vi "SVI_NewE2E_FindComPort.vi"(2 "Error In":errorcluster, 3 "ID to Match":string) -> (0 "error out":errorcluster, 1 "VISA resource name":refnum<visa-resource-name>)   [LabVIEW 2014]
uses:
  <vilib>/regexp/Match Regular Expression.xnode
panel:
  out "ID Message":string
  out "Responses":string[][](array[string])
  out "Attempts Taken":i32
  out "Current Check":refnum<visa-resource-name>
  out "COM only list":string[](array[string])
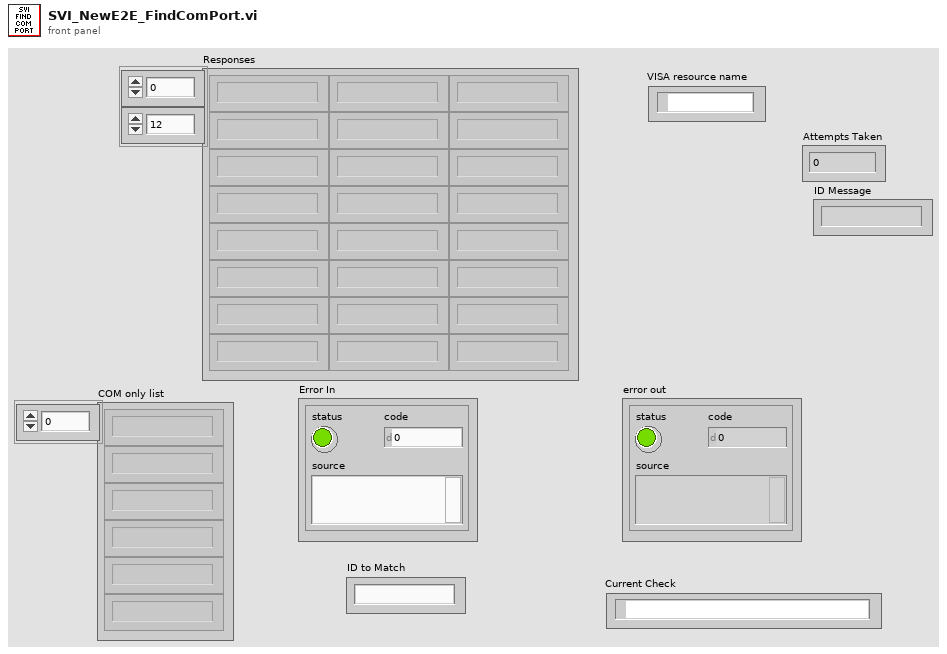
[diagram p1: front panel]
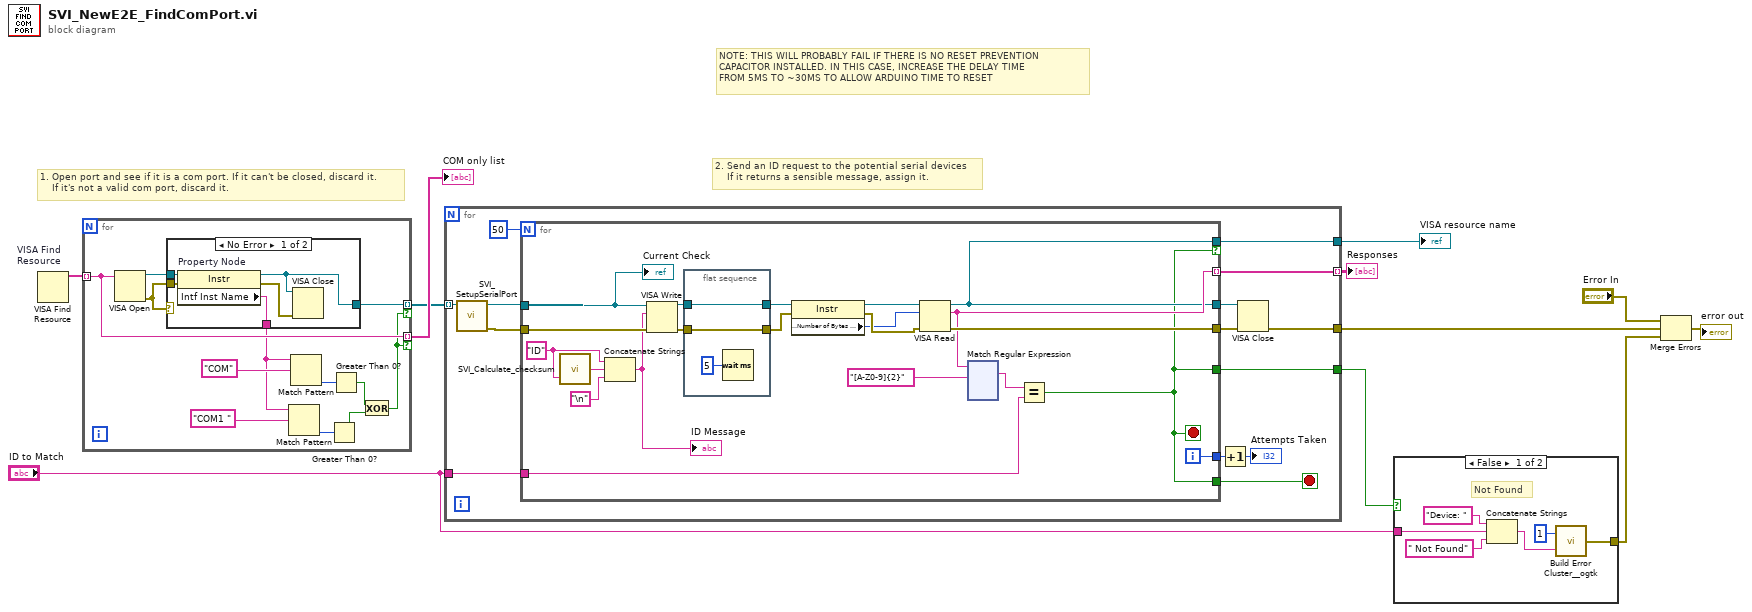
[diagram p0: block diagram]
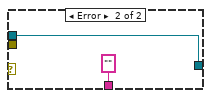
[diagram p2: hidden frame]
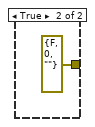
[diagram p3: hidden frame]
diagram:
  # "NOTE: THIS WILL PROBABLY FAIL IF THERE IS NO RESET PREVENTION\nCAPACITOR INSTALLED. IN THIS CASE, INCREASE THE DELAY TIME \nFROM 5MS TO ~30MS TO ALLOW ARDUINO TIME TO RESET"
  # "2. Send an ID request to the potential serial devices\n    If it returns a sensible message, assign it."
  # "1. Open port and see if it is a com port. If it can't be closed, discard it.\n    If it's not a valid com port, discard it."
  n1 = VISA Find Resource "VISA Find\nResource"() -> (3:w11:string[])  [unwired: 3 in, 2 out]
  n2 = for {
    tunnel: w11 -> [w20] mode=indexing
    tunnel: [w20] -> w10 mode=indexing if=w14
    tunnel: [w19] -> w9 mode=indexing if=w14
    n3 = VISA Open(VISA resource name=w20) -> (VISA resource name=w23:refnum<visa-resource-name>, error out=w12:errorcluster)  [unwired: 4 in]
    n4 = case shown="No Error" w12 {
      tunnel: w23 -> [w28 w30]
      tunnel: w12 -> [w27 _]
      tunnel: [w25 w30] -> w19
      tunnel: [w24 "" ("Intf Inst Name")] -> w13
      frame No Error {
        n5 = property on="Property Node" class="Instr"(reference=w28, error in=w27) -> (reference out=w25:refnum<visa-resource-name>, error out=w26:errorcluster, "Intf Inst Name"=w24:string)
        n6 = VISA Close(VISA resource name=w25, error in (no error)=w26) -> ()  [unwired: 1 out]
      }
      frame Error {
      }
    }
    n7 = Match Pattern(string=w13, regular expression="COM1 ") -> (offset past match=w18:i32)  [unwired: 1 in, 3 out]
    n8 = Match Pattern(string=w13, regular expression="COM") -> (offset past match=w21:i32)  [unwired: 1 in, 3 out]
    n9 = Greater Than 0?(x=w18) -> (x > 0?=w16:bool)
    n10 = Greater Than 0?(x=w21) -> (x > 0?=w15:bool)
    n11 = Exclusive Or(1:w16, 2:w15) -> (0:w14:bool)
  }
  "COM only list" <- w10
  n12 = for {
    tunnel: w9 -> [w39] mode=indexing
    tunnel: [w38] -> w5
    tunnel: [w37] -> w3 mode=indexing
    tunnel: [w36] -> w2
    tunnel: "ID to Match" -> [w33]
    tunnel: [w32] -> w8
    stop <- w34 stop-if-true
    n13 = call "SVI_SetupSerialPort.vi"("VISA Refnum in"=w39) -> ("error out"=w40:errorcluster, "VISA Refnum out"=w44:refnum<visa-resource-name>)  [unwired: 9 in]
    n14 = for {
      N: 50 -> [_]
      tunnel: w40 -> [w59]
      tunnel: w44 -> [w54]
      tunnel: [w57] -> w42
      tunnel: [w49] -> w41
      tunnel: [w55] -> w35
      tunnel: [w53] -> w37 mode=indexing
      tunnel: [w49] -> w36 if=w46
      tunnel: [w46] -> w34
      tunnel: w33 -> [w47]
      tunnel: [w46] -> w32
      i -> [w55]
      stop <- w46 stop-if-true
      w51 = "ID" ("write buffer")
      n15 = call "SVI_Calculate_checksum.vi"("Message"=w51) -> ("Calculated checksum"=w52:string)  [unwired: 1 in]
      n16 = Concatenate Strings(w51, w52, "\n") -> (w45:string)
      "ID Message" <- w45
      n17 = VISA Write(VISA resource name=w54, write buffer=w45, error in (no error)=w59) -> (VISA resource name out=w61:refnum<visa-resource-name>, error out=w60:errorcluster)  [unwired: 1 out]
      n18 = flat-sequence {
        tunnel: [w181] -> w62
        tunnel: w61 -> [w181]
        tunnel: [w180] -> w63
        tunnel: w60 -> [w180]
        frame #0 {
          n19 = Wait (ms)(milliseconds to wait=u32 5) -> ()  [unwired: 1 out]
        }
      }
      n20 = property class="Instr"(reference=w62, error in=w63) -> (reference out=w65:refnum<visa-resource-name>, error out=w64:errorcluster, "Serial Settings:Number of Bytes at Serial Port"=w56:u32)
      n21 = VISA Read(VISA resource name=w65, byte count=w56, error in (no error)=w64) -> (VISA resource name out=w49:refnum<visa-resource-name>, read buffer=w53:string, error out=w57:errorcluster)  [unwired: 1 out]
      n22 = xnode "Match Regular Expression"("input string"=w53, "regular expression"="[A-Z0-9]{2}") -> ("whole match"=w48:string)  [unwired: 4 in, 4 out]
      n23 = Equal?(x=w48, y=w47) -> (x = y?=w46:bool)
      "Current Check" <- w54
    }
    n24 = Increment(x=w35) -> (x+1=→"Attempts Taken":i32)
    n25 = VISA Close(VISA resource name=w41, error in (no error)=w42) -> (error out=w38:errorcluster)
  }
  "Responses" <- w3
  "VISA resource name" <- w2
  n26 = case shown="False" w8 {
    tunnel: [w187 errorcluster {"status"=FALSE, "code"=0, "source"=""} ("error out")] -> w6
    tunnel: "ID to Match" -> [w183 _]
    frame False {
      # "Not Found"
      n27 = Concatenate Strings("Device: " ("string"), w183, " Not Found" ("String to Prepend to source (\"\")")) -> (w185:string)
      n28 = call <userlib>:"Build Error Cluster__ogtk.vi"("String to Prepend to source (\"\")"=w185, "code"=1) -> ("error out"=w187:errorcluster)
    }
    frame True {
    }
  }
  n29 = Merge Errors("Error In", w5, w6) -> (→"error out":errorcluster)
